vi "main.vi"() -> ()   [LabVIEW 2020, in "Approach Curve.lvclass"]
uses:
  Approach Curve.lvclass
  Approach Curve.lvclass/Approach Curve.ctl
panel:
  in  "Tab Control":enum32{"Page 1", "Page 2"}(tab)
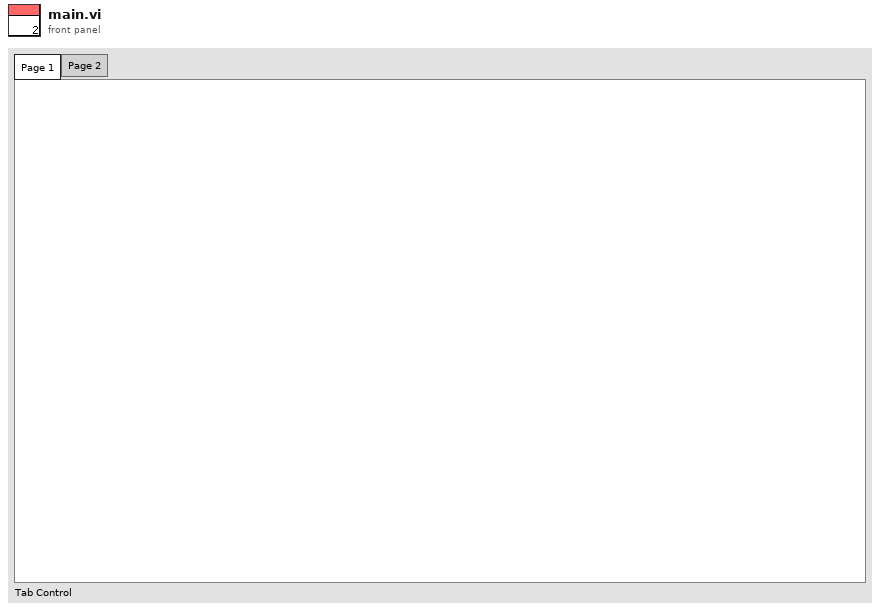
[diagram p1: front panel]
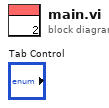
[diagram p0: block diagram]
diagram:
